vi "home with centering offset.vi"   [LabVIEW 2010]
panel:
  # "homes motor\n+offset"
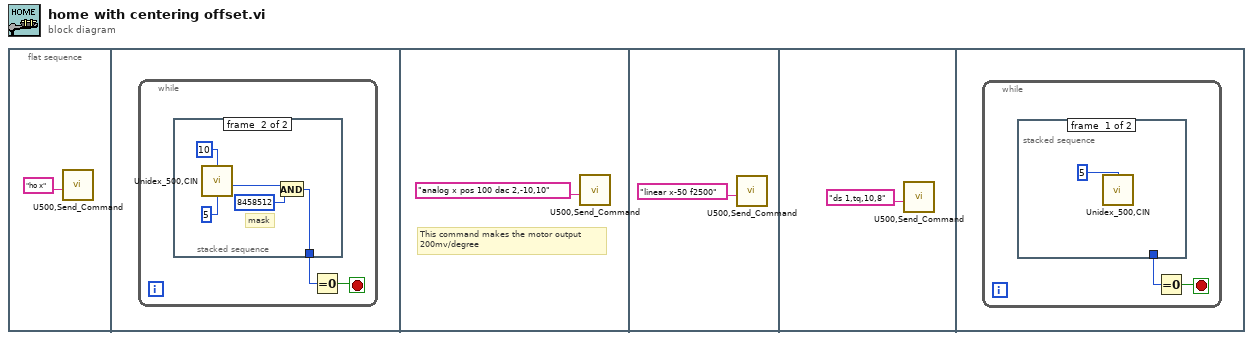
[diagram p0: block diagram]
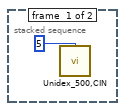
[diagram p2: hidden frame]
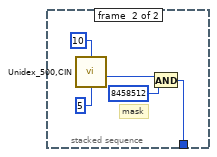
[diagram p3: hidden frame]
diagram:
  n1 = flat-sequence {
    frame #0 {
      n2 = call "U500,Send_Command.vi"("Command String"="ho x") -> ()  [unwired: 9 in, 2 out]
    }
    frame #1 {
      n3 = while {
        stop <- w3 stop-if-true
        n4 = stacked-sequence {
          tunnel: [_ w5] -> w2
          frame #0 {
            n5 = call "Unidex_500,CIN.VI"("Library Function"=5) -> ()  [unwired: 5 in, 4 out]
          }
          frame #1 {
            # "mask"
            n6 = call "Unidex_500,CIN.VI"("Library Function"=10, "int which"=i16 5) -> ("Status"=w6:u32)  [unwired: 4 in, 3 out]
            n7 = And(x=w6, y=8458512) -> (x .and. y?=w5:u32)
          }
        }
        n8 = Equal To 0?(x=w2) -> (x = 0?=w3:bool)
      }
    }
    frame #2 {
      # "This command makes the motor output\n200mv/degree"
      n9 = call "U500,Send_Command.vi"("Command String"="analog x pos 100 dac 2,-10,10") -> ()  [unwired: 9 in, 2 out]
    }
    frame #3 {
      n10 = call "U500,Send_Command.vi"("Command String"="linear x-50 f2500") -> ()  [unwired: 9 in, 2 out]
    }
    frame #4 {
      n11 = call "U500,Send_Command.vi"("Command String"="ds 1,tq,10,8") -> ()  [unwired: 9 in, 2 out]
    }
    frame #5 {
      n12 = while {
        stop <- w14 stop-if-true
        n13 = stacked-sequence {
          tunnel: [_ w16] -> w13
          frame #0 {
            n14 = call "Unidex_500,CIN.VI"("Library Function"=5) -> ()  [unwired: 5 in, 4 out]
          }
          frame #1 {
            # "mask"
            n15 = call "Unidex_500,CIN.VI"("Library Function"=10, "int which"=i16 5) -> ("Status"=w17:u32)  [unwired: 4 in, 3 out]
            n16 = And(x=w17, y=8458512) -> (x .and. y?=w16:u32)
          }
        }
        n17 = Equal To 0?(x=w13) -> (x = 0?=w14:bool)
      }
    }
  }
